vi "Get Exit Code.vi"(8 "error in":errorcluster, 10 "ignore error if process running (T)":bool=TRUE, 11 "pipe in":T1) -> (0 "error out":errorcluster, 1 "not running?":bool, 2 "exit code":i32, 3 "pipe out":T1, 4 "exited?":bool)   [LabVIEW 2020, in "LV Process library.lvlib"]
doc: "Calls lv_proc.dll and reads process exit code. Error is returned if process has not exited yet. Optionally this error can be filtered by 'ignore error if still active' (default), thus one can find out if process is still running.\n\nOutput terminals:\n\"<b>exited?</b>\" is true if process returned exit code (exited) but process handles are still opened and valid. If true, call cleanup VI as soon as possible to close the process handles.\n\"<b>not running?</b>\" is true if process exited or process handles not passed or not valid.\n\n---\nLV Process works only with lv_proc.dll library, which is part of vipm package or should be delivered together with packed library. Placement of this dll is selected in terminal of Create Process.vi."
uses:
  LV Process library.lvlib
  Pipe Handle.ctl
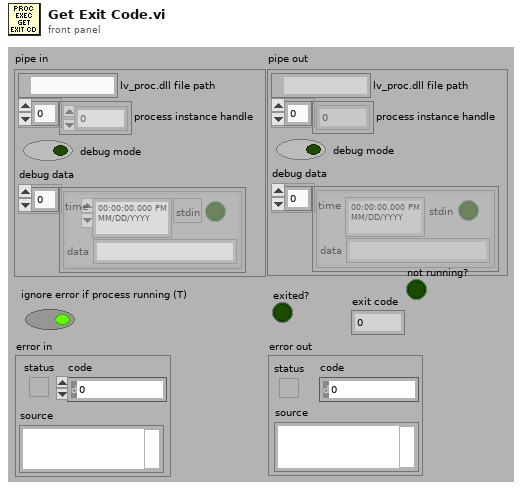
[diagram p1: front panel]
types:
  T1 = typedef "LV Process library.lvlib/Pipe Handle.ctl" = cluster{"lv_proc.dll file path":path, "process instance handle":u32[], "debug mode":bool, "debug data":cluster{"time":timestamp, "stdin":bool, "data":string}[]}
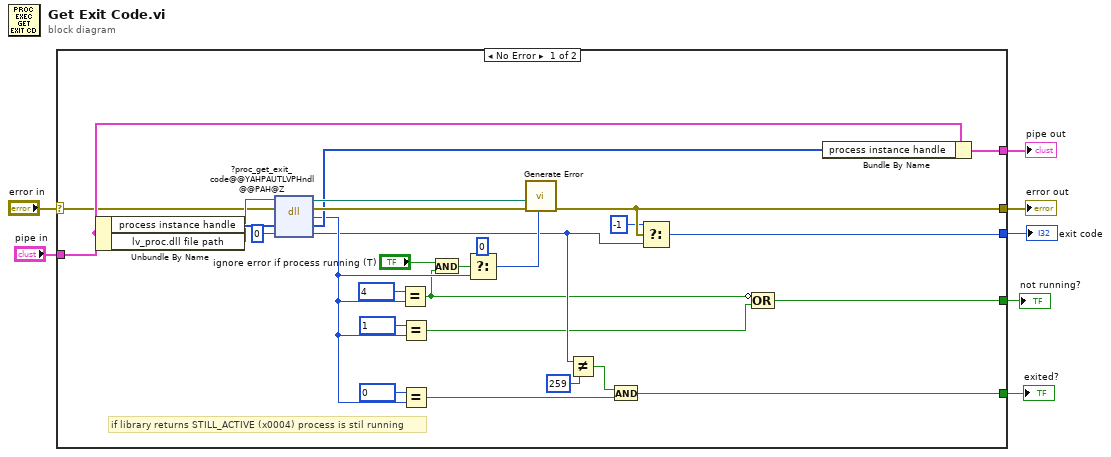
[diagram p0: block diagram]
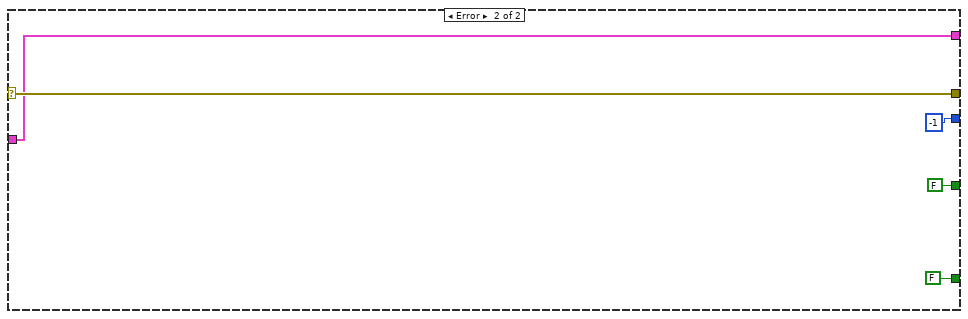
[diagram p2: hidden frame]
diagram:
  n1 = case shown="No Error" "error in" {
    selector: "error in" -> [w25 w40]
    tunnel: "pipe in" -> [w31 w39]
    tunnel: [w21 w40] -> w6
    tunnel: [w24 w39] -> w4
    tunnel: [w8 FALSE] -> w3
    tunnel: [w19 -1 ("code")] -> w2
    tunnel: [w9 FALSE] -> w1
    frame No Error {
      # "if library returns STILL_ACTIVE (x0004) process is stil running"
      n2 = Unbundle By Name(w31) -> ("process instance handle"=w33:u32[], "lv_proc.dll file path"=w32:path)
      n3 = dll-call lib="C:/Data/GOLPI/LV Process/lv_proc.dll" fn="?proc_get_exit_code@@YAHPAUTLVPHndl@@PAH@Z" label="proc_get_exit_code"(path in=w32, error in=w25, "proc"=w33, "code"=0 ("code mem")) -> (path out=w27:path, error out=w28:errorcluster, "error"=w15:i32, "proc"=w26:u32[], "code"=w13:i32)  [unwired: 1 in]
      n4 = Equal?(x=4, y=w15) -> (x = y?=w11:bool)
      n5 = Equal?(x=1, y=w15) -> (x = y?=w10:bool)
      n6 = Equal?(x=0, y=w15) -> (x = y?=w17:bool)
      n7 = And(x="ignore error if process running (T)", y=w11) -> (x .and. y?=w23:bool)
      n8 = Select(t=0, s=w23, f=w15) -> (s? t:f=w29:i32)
      n9 = call "Generate Error.vi"("error code in"=w29, "error in"=w28, "lv_proc.dll path in"=w27) -> ("error out"=w21:errorcluster)  [unwired: 6 in, 1 out]
      n10 = Not Equal?(x=w13, y=259) -> (x != y?=w12:bool)
      n11 = And(x=w12, y=w17) -> (x .and. y?=w8:bool)
      n12 = Select(t=-1, s=w21, f=w13) -> (s? t:f=w19:i32)
      n13 = Compound Arithmetic op=OR(invert w11, w10) -> (w9:bool)
      n14 = Bundle By Name(cluster=w31, "process instance handle"=w26) -> (w24:T1)
    }
    frame Error {
    }
  }
  "error out" <- w6
  "pipe out" <- w4
  "exited?" <- w3
  "exit code" <- w2
  "not running?" <- w1
